vi "Set Visible State on Multiple Controls.vi"(8 "error in (no error)":errorcluster, 10 "Visible?":bool, 11 "Controls":refnum<vi>[](array[refnum])) -> (0 "error out":errorcluster)   [LabVIEW 2026]
doc: "Sets all the controls in the input array to the \"Enable state\" value."
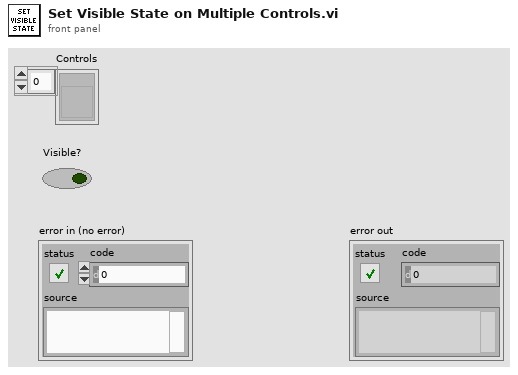
[diagram p1: front panel]
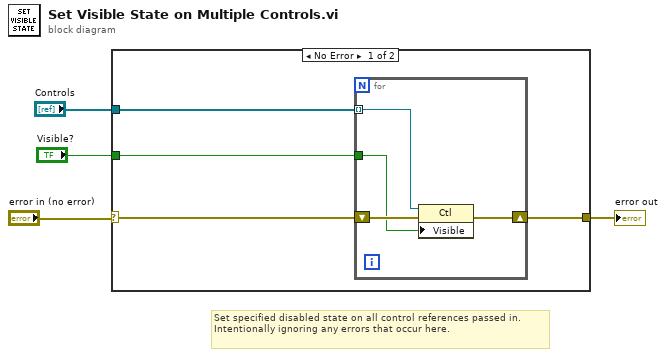
[diagram p0: block diagram]
diagram:
  # "Set specified disabled state on all control references passed in. Intentionally ignoring any errors that occur here."
  n1 = case shown="No Error" "error in (no error)" {
    selector: "error in (no error)" -> [w7 w13]
    tunnel: "Controls" -> [w8 _]
    tunnel: "Visible?" -> [w5 _]
    tunnel: [w6 w13] -> w1
    frame No Error {
      n2 = for {
        tunnel: w8 -> [w12] mode=indexing
        shift-right: [w10] -> w6
        shift-left: w7 -> [w11]
        tunnel: w5 -> [w9]
        n3 = property class="Ctl"(reference=w12, error in=w11, "Visible"=w9) -> (error out=w10:errorcluster)  [unwired: 1 out]
      }
    }
    frame Error {
    }
  }
  "error out" <- w1
